vi "Soft Start.vi"(0 "X- axis Joystick":dbl(slide) scale=-1.0..1.0, 1 "Z-axis Joystick":dbl(slide) scale=-1.0..1.0, 2 "X-Slew Rate":dbl=0.05, 3 "Y-Slew Rate":dbl=0.05, 4 "Z-Slew Rate":dbl=0.05, 5 "Y-axis Joystick":dbl(slide) scale=-1.0..1.0) -> (6 "X-axis drive":dbl, 7 "Z-axis drive":dbl, 8 "Y-axis drive":dbl)   [LabVIEW 2015]
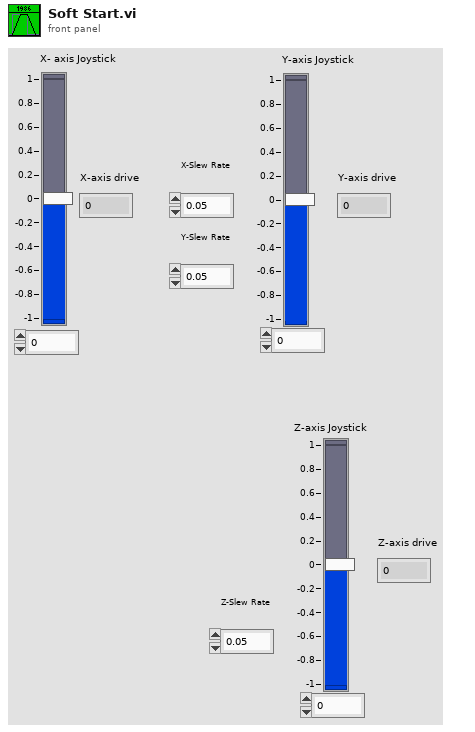
[diagram p1: front panel]
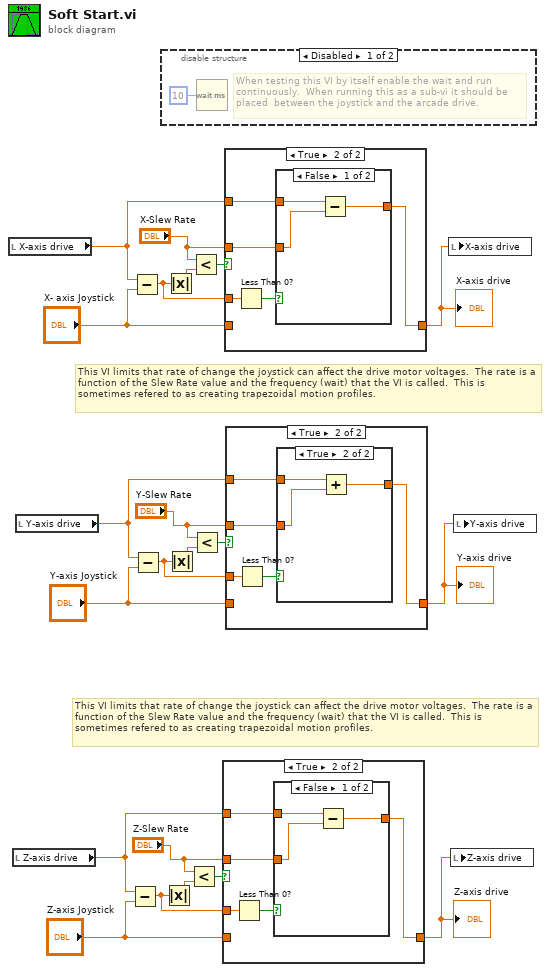
[diagram p0: block diagram]
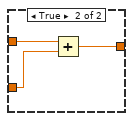
[diagram p3: hidden frame]
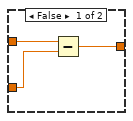
[diagram p6: hidden frame]
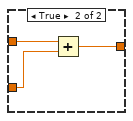
[diagram p8: hidden frame]
diagram:
  # "This VI limits that rate of change the joystick can affect the drive motor voltages.  The rate is a function of the Slew Rate value and the frequency (wait) that the VI is called.  This is sometimes refered to as creating trapezoidal motion profiles."
  # "This VI limits that rate of change the joystick can affect the drive motor voltages.  The rate is a function of the Slew Rate value and the frequency (wait) that the VI is called.  This is sometimes refered to as creating trapezoidal motion profiles."
  n1 = local read "X-axis drive"() -> (w16:dbl)
  n2 = local read "Z-axis drive"() -> (w2:dbl)
  n3 = local read "Y-axis drive"() -> (w10:dbl)
  n4 = Subtract(x=w2, y="Z-axis Joystick") -> (x-y=w4:dbl)
  n5 = Subtract(x=w16, y="X- axis Joystick") -> (x-y=w18:dbl)
  n6 = Subtract(x=w10, y="Y-axis Joystick") -> (x-y=w12:dbl)
  n7 = disable-structure shown="Disabled" {
    frame Disabled {
      # "When testing this VI by itself enable the wait and run continuously.  When running this as a sub-vi it should be placed  between the joystick and the arcade drive."
      n8 = Wait (ms)(milliseconds to wait=u32 10) -> ()  [unwired: 1 out]
    }
    frame Enabled {
    }
  }
  n9 = Absolute Value(x=w4) -> (abs(x)=w7:dbl)
  n10 = Absolute Value(x=w18) -> (abs(x)=w21:dbl)
  n11 = Absolute Value(x=w12) -> (abs(x)=w15:dbl)
  n12 = Less?(x="Z-Slew Rate", y=w7) -> (x < y?=w6:bool)
  n13 = Less?(x="X-Slew Rate", y=w21) -> (x < y?=w20:bool)
  n14 = Less?(x="Y-Slew Rate", y=w15) -> (x < y?=w14:bool)
  n15 = case shown="True" w6 {
    tunnel: [w23 w24] -> w3
    tunnel: "Z-axis Joystick" -> [w23 _]
    tunnel: w4 -> [_ w28]
    tunnel: w2 -> [_ w26]
    tunnel: "Z-Slew Rate" -> [_ w25]
    frame False {
    }
    frame True {
      n16 = Less Than 0?(x=w28) -> (x < 0?=w27:bool)
      n17 = case shown="False" w27 {
        tunnel: w26 -> [w31 w34]
        tunnel: w25 -> [w29 w32]
        tunnel: [w30 w33] -> w24
        frame False {
          n18 = Subtract(x=w31, y=w29) -> (x-y=w30:dbl)
        }
        frame True {
          n19 = Add(x=w34, y=w32) -> (x+y=w33:dbl)
        }
      }
    }
  }
  "Z-axis drive" <- w3
  n20 = case shown="True" w20 {
    tunnel: [w35 w36] -> w17
    tunnel: "X- axis Joystick" -> [w35 _]
    tunnel: w18 -> [_ w40]
    tunnel: w16 -> [_ w38]
    tunnel: "X-Slew Rate" -> [_ w37]
    frame False {
    }
    frame True {
      n21 = Less Than 0?(x=w40) -> (x < 0?=w39:bool)
      n22 = case shown="False" w39 {
        tunnel: w38 -> [w43 w46]
        tunnel: w37 -> [w41 w44]
        tunnel: [w42 w45] -> w36
        frame False {
          n23 = Subtract(x=w43, y=w41) -> (x-y=w42:dbl)
        }
        frame True {
          n24 = Add(x=w46, y=w44) -> (x+y=w45:dbl)
        }
      }
    }
  }
  "X-axis drive" <- w17
  n25 = case shown="True" w14 {
    tunnel: [w47 w48] -> w11
    tunnel: "Y-axis Joystick" -> [w47 _]
    tunnel: w12 -> [_ w52]
    tunnel: w10 -> [_ w50]
    tunnel: "Y-Slew Rate" -> [_ w49]
    frame False {
    }
    frame True {
      n26 = Less Than 0?(x=w52) -> (x < 0?=w51:bool)
      n27 = case shown="True" w51 {
        tunnel: w50 -> [w55 w58]
        tunnel: w49 -> [w53 w56]
        tunnel: [w54 w57] -> w48
        frame False {
          n28 = Subtract(x=w55, y=w53) -> (x-y=w54:dbl)
        }
        frame True {
          n29 = Add(x=w58, y=w56) -> (x+y=w57:dbl)
        }
      }
    }
  }
  "Y-axis drive" <- w11
  n30 = local write "X-axis drive"(w17) -> ()
  n31 = local write "Z-axis drive"(w3) -> ()
  n32 = local write "Y-axis drive"(w11) -> ()
